vi "Fpga-Uart-Exercisor.vi"() -> ()   [LabVIEW 2017]
panel:
  out "gpio_rtl_0_tri_o":u32
  in  "reset_rtl":bool
  in  "gpio_rtl_tri_i":u32
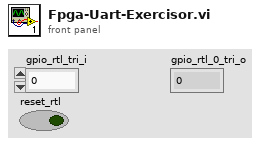
[diagram p1: front panel]
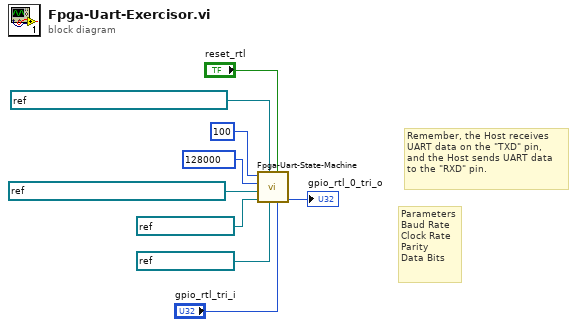
[diagram p0: block diagram]
diagram:
  w8 = u32 128000 items=["110"=110, "300"=300, "1200"=1200, "2400"=2400, "4800"=4800, "9600"=9600, "19200"=19200, "38400"=38400, "57600"=57600, "115200"=115200, "128000"=128000, "230400"=230400, "460800"=460800, "921600"=921600] ("Baud Rate")
  # "Parameters\nBaud Rate\nClock Rate\nParity\nData Bits"
  # "Remember, the Host receives\nUART data on the \"TXD\" pin,\nand the Host sends UART data\nto the \"RXD\" pin."
  n1 = call "Fpga-Uart-State-Machine.vi"("gpio_rtl_tri_i"="gpio_rtl_tri_i", "reset_rtl"="reset_rtl", "TX FIFO In"=refnum<k21> "HT-UART_TX", "RXD Pin In"=refnum<k21> "UserRTL_d_microblaze_i\\uart_rtl_rxd", "RX FIFO In"=refnum<k21> "TH-UART_RX", "TXD Pin In"=refnum<k21> "UserRTL_d_microblaze_i\\uart_rtl_txd", "Baud Rate"=w8, "FPGA Clock Rate (MHz)"=u32 100) -> ("gpio_rtl_0_tri_o"=→"gpio_rtl_0_tri_o":u32)  [unwired: 3 in]
